vi "Save to TDMS Core.vi"(8 "Error In":errorcluster, 10 "TDMS Ref":refnum<k34>, 11 "LHW-DataCollection in":refnum<class "LHW-DataCollection.lvclass">) -> (0 "Error Out":errorcluster, 3 "LHW-DataCollection out":refnum<class "LHW-DataCollection.lvclass">)   [LabVIEW 2016, in "LHW-Data.lvlib" / "LHW-DataCollection.lvclass"]
doc: "Save data to TDMS file."
uses:
  LHW-DataCollection.lvclass
  LHW-DataCollection.lvclass/LHW-DataCollection.ctl
  Read LHW-Data Objects.vi
  LHW-Data/LHW-Data.lvclass
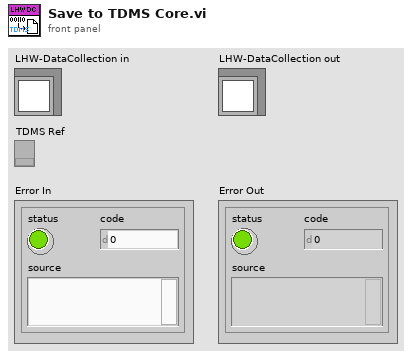
[diagram p1: front panel]
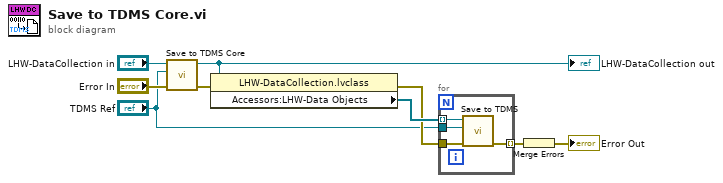
[diagram p0: block diagram]
diagram:
  n1 = call-parent "Save to TDMS Core.vi"("Error In"="Error In", "TDMS Ref"="TDMS Ref", "LHW-Data in"="LHW-DataCollection in") -> ("Error Out"=w6:errorcluster, "LHW-Data out"=w7:refnum<class "LHW-DataCollection.lvclass">)  [unwired: 7 in]
  "LHW-DataCollection out" <- w7
  n2 = property class="LHW-DataCollection.lvclass"(reference=w7, error in=w6) -> (error out=w4:errorcluster, "Accessors:LHW-Data Objects"=w5:refnum<class "LHW-Data.lvclass">[])  [unwired: 1 out]
  n3 = for {
    tunnel: w5 -> [w13] mode=indexing
    tunnel: w4 -> [w12]
    tunnel: "TDMS Ref" -> [w11]
    tunnel: [w10] -> w2 mode=indexing
    n4 = call "Save to TDMS.vi"("Error In"=w12, "TDMS Ref"=w11, "LHW-Data in"=w13) -> ("Error Out"=w10:errorcluster)  [unwired: 7 in, 1 out]
  }
  n5 = Merge Errors(w2) -> (→"Error Out":errorcluster)
